vi "init.vi"(8 "error in":errorcluster, 10 "TBM module configuration in":refnum<class "TBM module configuration.lvclass">, 11 "Modbus Slave runtime in":refnum<class "Modbus Slave runtime.lvclass">) -> (0 "error out":errorcluster, 1 "data allocations":T1, 2 "execution settings":T4, 3 "Modbus Slave runtime out":refnum<class "Modbus Slave runtime.lvclass">)   [LabVIEW 2013, in "Modbus Slave runtime.lvclass"]
doc: "Provides an interface for initializing a module at runtime. While this interface performs no operations, a child should provide an override which may open any necessary references or sessions, allocate necessary memory, and perform any final configuration validataion before providing the full configuration <b>execution data</b> to the calling process.Platypus Framework 1.0.1.65\nNI Systems Engineering - National Instruments"
uses:
  Modbus Slave runtime.lvclass
  <vilib>/NI/Tag Bus Module Framework/module configuration/TBM module configuration.lvclass
  <vilib>/NI/Tag Bus Module Framework/runtime/execution settings.ctl
  <vilib>/NI/Tag Bus Module Framework/channel/data tables.ctl
  <vilib>/NI/Tag Bus/dictionary/data dictionary.lvclass
  <vilib>/NI/Tag Bus/dictionary table pair.ctl
  <vilib>/NI/Tag Bus/table/data table.ctl
  configuration/Modbus Slave configuration.lvclass
  configuration/Modbus Slave configuration.lvclass/Modbus Slave configuration.ctl
  Modbus Slave runtime.lvclass/Modbus Slave runtime.ctl
  configuration/Read port (502).vi
  configuration/Read modbus channels.vi
  <vilib>/NI/Modbus Library/API/Wrapper/Create TCP Slave.vi
  module channel/Modbus Module Channel.lvclass
  <vilib>/NI/Tag Bus Module Framework/channel/TBM channel.lvclass
  <vilib>/NI/Tag Bus Module Framework/runtime/TBM module execution interface.lvclass
  <vilib>/NI/Modbus Library/API/Wrapper/API Main.lvlib
  <vilib>/NI/Tag Bus/tag bus.lvlib
  <vilib>/NI/Tag Bus/table/data table.lvlib
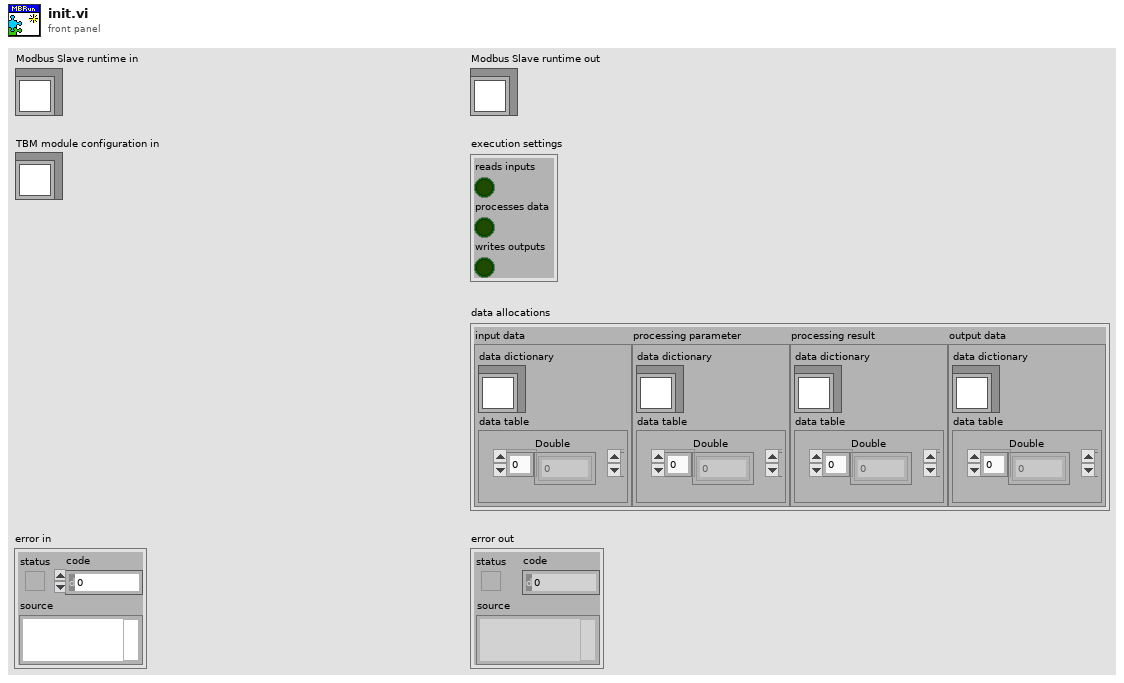
[diagram p1: front panel]
types:
  T1 = typedef "TBM channel.lvclass/data tables.ctl" = cluster{"input data":T2, "processing parameter":T2, "processing result":T2, "output data":T2}
  T2 = typedef "tag bus.lvlib/dictionary table pair.ctl" = cluster{"data dictionary":refnum<class "data dictionary.lvclass">, "data table":T3}
  T3 = typedef "tag bus.lvlib/data table.lvlib/data table.ctl" = cluster{"Double":dbl[], "Single":sgl[], "I64":i64[], "I32":i32[], "I16":i16[], "I8":i8[], "U64":u64[], "U32":u32[], "U16":u16[], "U8":u8[], "Boolean":bool[], "String":string[], "Array of Double":cluster{"DBL Array":dbl[]}[], "Array of Single":cluster{"SGL Array":sgl[]}[], "Array of I64":cluster{"I64 Array":i64[]}[], "Array of I32":cluster{"I32 Array":i32[]}[], "Array of I16":cluster{"I16 Array":i16[]}[], "Array of I8":cluster{"I8 Array":i8[]}[], "Array of U64":cluster{"U64 Array":u64[]}[], "Array of U32":cluster{"U32 Array":u32[]}[], "Array of U16":cluster{"U16 Array":u16[]}[], "Array of U8":cluster{"U8 Array":u8[]}[], "Array of Boolean":cluster{"Boolean Array":bool[]}[], "Array of String":cluster{"String Array":string[]}[]}
  T4 = typedef "TBM module execution interface.lvclass/execution settings.ctl" = cluster{"reads inputs":bool, "processes data":bool, "writes outputs":bool}
  T5 = typedef "Modbus Slave runtime.lvclass/output bulk data access.ctl" = cluster{"modbus type":T6, "start":u16, "length":u16, "maps":T7[], "coils":bool[], "registers":u16[]}
  T6 = typedef "Modbus Module Channel.lvclass/data bank type.ctl" = enum16{"coils", "discrete inputs", "input registers", "holding registers"}
  T7 = typedef "Modbus Slave runtime.lvclass/data mapping elements.ctl" = cluster{"data type":T8, "data index":i32, "element index":i32, "subindex":i32}
  T8 = typedef "tag bus.lvlib/tag descriptor.lvclass/Data Type.ctl" = enum16{"Double", "Single", "I64", "I32", "I16", "I8", "U64", "U32", "U16", "U8", "Boolean", "String", "Array of Double", "Array of Single", "Array of I64", "Array of I32", "Array of I16", "Array of I8", "Array of U64", "Array of U32", "Array of U16", "Array of U8", "Array of Boolean", "Array of String"}
  T9 = typedef "Modbus Slave runtime.lvclass/bulk data access.ctl" = cluster{"modbus type":T6, "start":u16, "length":u16, "maps":T7[]}
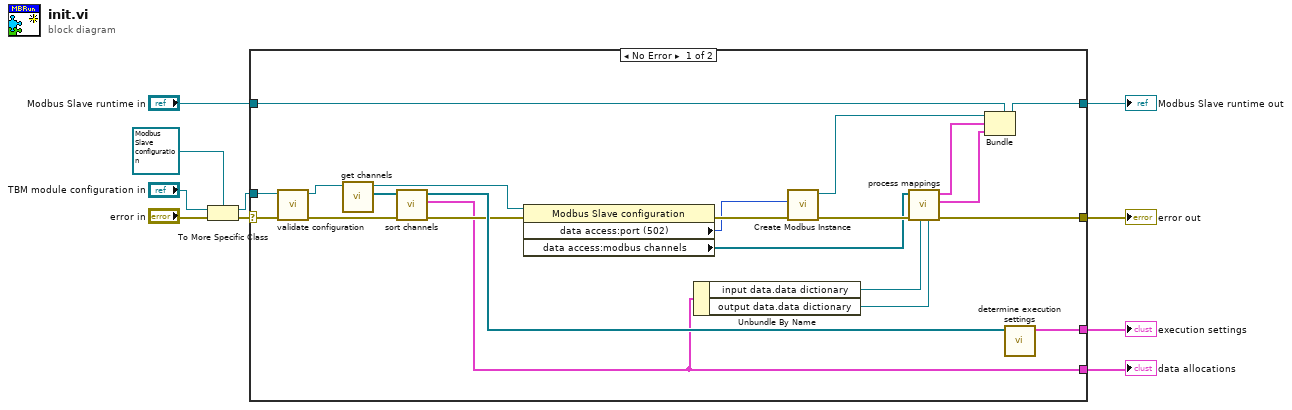
[diagram p0: block diagram]
diagram:
  n1 = To More Specific Class(target class=refnum<class "Modbus Slave configuration.lvclass"> refnum ("Synchronous module configuration"), reference="TBM module configuration in", error in="error in") -> (specific class reference=w9:refnum<class "Modbus Slave configuration.lvclass">, error out=w10:errorcluster)
  n2 = case shown="No Error" w10 {
    selector: w10 -> [w28 w33]
    tunnel: w9 -> [w27 _]
    tunnel: "Modbus Slave runtime in" -> [w32 w34]
    tunnel: [w24 w34] -> w4
    tunnel: [w15 w33] -> w3
    tunnel: [w16 _] -> w1
    tunnel: [w31 _] -> w2
    frame No Error {
      n3 = call-dynamic "validate configuration.vi"("error in"=w28, "Modbus Slave configuration in"=w27) -> ("error out"=w29:errorcluster, "Modbus Slave configuration out"=w26:refnum<class "Modbus Slave configuration.lvclass">)  [unwired: 8 in]
      n4 = call-dynamic "get channels.vi"("Modbus Slave configuration in"=w26) -> ("channels"=w25:refnum<class "TBM channel.lvclass">[], "Modbus Slave configuration out"=w20:refnum<class "Modbus Slave configuration.lvclass">)  [unwired: 9 in]
      n5 = call <vilib>:"sort channels.vi"("error in"=w29, "channels in"=w25) -> ("error out"=w23:errorcluster, "data allocations"=w16:T1, "channels out"=w30:refnum<class "TBM channel.lvclass">[])  [unwired: 7 in]
      n6 = property class="Modbus Slave configuration"(reference=w20, error in=w23) -> (error out=w21:errorcluster, "data access:port (502)"=w19:u16, "data access:modbus channels"=w11:refnum<class "Modbus Module Channel.lvclass">[])  [unwired: 1 out]
      n7 = Unbundle By Name(w16) -> ("input data.data dictionary"=w13:refnum<class "data dictionary.lvclass">, "output data.data dictionary"=w12:refnum<class "data dictionary.lvclass">)
      n8 = call-poly <vilib>:"Create Modbus Instance.vi"("error in"=w21, "port (502)"=w19) -> ("error out"=w14:errorcluster, "TCP slave instance"=w22:refnum<class "Modbus Slave.lvclass">)  [unwired: 8 in]
      n9 = call "process mappings.vi"("output dictionary"=w12, "input dictionary"=w13, "error in"=w14, "modbus channels"=w11) -> ("error out"=w15:errorcluster, "output accesses"=w18:T5[], "input accesses"=w17:T9[])  [unwired: 5 in]
      n10 = Bundle(cluster=w32, w22, w17, w18) -> (w24:refnum<class "Modbus Slave runtime.lvclass">)
      n11 = call <vilib>:"determine execution settings.vi"("channels"=w30) -> ("execution settings"=w31:T4)  [unwired: 10 in]
    }
    frame Error {
    }
  }
  "error out" <- w3
  "Modbus Slave runtime out" <- w4
  "execution settings" <- w2
  "data allocations" <- w1
